vi "LVClass_WavefrontCorrectorSet ctor from WavefrontCorrector.vi"(0 "WavefrontCorrectorSet (const)":refnum<class "WavefrontCorrectorSet.lvclass">, 5 "WavefrontCorrectorSet":refnum<class "WavefrontCorrector.lvclass">, 11 "error in (no error)":errorcluster) -> (4 "WavefrontCorrectorSet (new)":refnum<class "WavefrontCorrectorSet.lvclass">, 6 "WavefrontCorrectorSet (dup)":refnum<class "WavefrontCorrector.lvclass">, 15 "error out":errorcluster)   [LabVIEW 2020, in "WavefrontCorrectorSet.lvclass"]
doc: "WavefrontCorrectorSet constructor.\n\n--------------------------------------------------------------------------------\n\n<B>wavefrontcorrector_setIn </B> : Constant Pointer to WavefrontCorrectorSet object.\n<B>wavefrontcorrector_setOut </B> : Constant Pointer to WavefrontCorrectorSet object.\n<B>config_file_path </B> : Absolute path to Haso or Camera configuration file.\n<B>ErrorIn </B> : Error\n<B>ErrorOut </B> : Error\n\n--------------------------------------------------------------------------------"
uses:
  WavefrontCorrectorSet.lvclass
  WavefrontCorrector.lvclass
  Handle creation.ctl
  WavefrontCorrectorSet.lvclass/WavefrontCorrectorSet.ctl
  LVClass_WavefrontCorrector Read WavefrontCorrector.vi
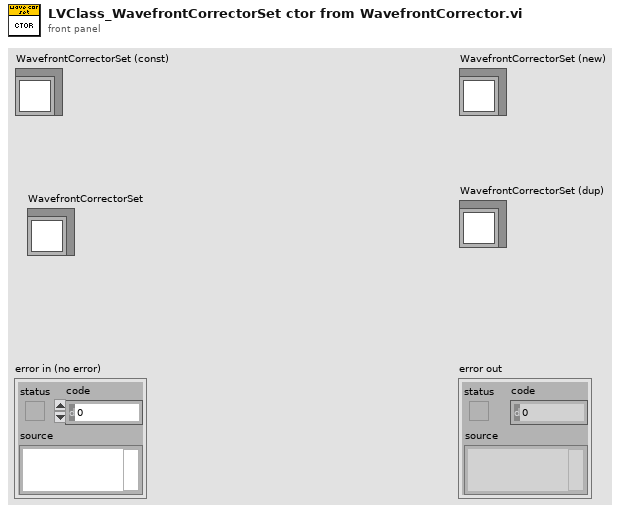
[diagram p1: front panel]
types:
  T1 = typedef "Handle creation.ctl" = enum16{"By ctor", "By write function"}
  T2 = typedef "ClassID.ctl" = i64
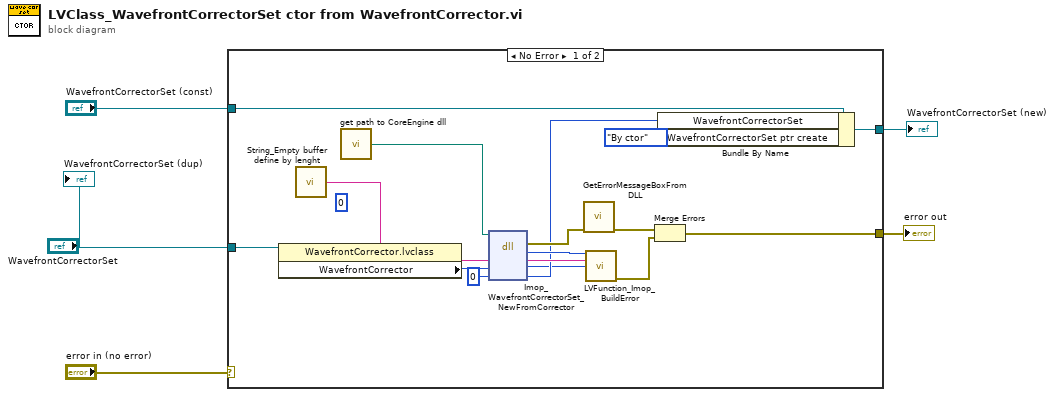
[diagram p0: block diagram]
diagram:
  n1 = case shown="No Error" "error in (no error)" {
    selector: "error in (no error)" -> [_ w23]
    tunnel: [w13 w23] -> w2
    tunnel: [w16 w22] -> w3
    tunnel: "WavefrontCorrectorSet (const)" -> [w17 w22]
    tunnel: "WavefrontCorrectorSet" -> [w11 _]
    frame No Error {
      (unwired) 0 ("Pupil")
      n2 = property class="WavefrontCorrector.lvclass"(reference=w11) -> ("WavefrontCorrector"=w9:T2)  [unwired: 1 in, 2 out]
      n3 = call "String_Empty buffer define by lenght.vi"() -> ("Empty buffer"=w10:string)  [unwired: 1 in]
      n4 = call "get path to CoreEngine dll.vi"() -> ("path to wavekit library"=w12:path)  [unwired: 14 in, 1 out]
      n5 = dll-call lib="D:/soft/HASO_v3/SVN_trunk/ImOpCoreEngine4_LV2011/DLLs/c_interface_vc100.dll" fn="Imop_WavefrontCorrectorSet_NewFromCorrector"(path in=w12, "message"=w10, "WavefrontCorrector"=w9, "WavefrontCorrectorSet"=i64 0) -> (error out=w19:errorcluster, "return type"=w20:i32, "message"=w21:string, "WavefrontCorrector"=w6:i64, "WavefrontCorrectorSet"=w8:i64)  [unwired: 2 in, 1 out]
      n6 = call "GetErrorMessageBoxFromDLL.vi"("error IN"=w19) -> ("error OUT"=w15:errorcluster)  [unwired: 10 in]
      n7 = call "LVFunction_Imop_BuildError.vi"("code"=w20, "String to Prepend to source (\"\")"=w21, "Adresse"=w6) -> ("error out"=w14:errorcluster)  [unwired: 12 in]
      n8 = Merge Errors(w15, w14) -> (w13:errorcluster)
      n9 = Bundle By Name(cluster=w17, "WavefrontCorrectorSet"=w8, "WavefrontCorrectorSet ptr create"=Handle_creation."By ctor" ("Pupil ptr create")) -> (w16:refnum<class "WavefrontCorrectorSet.lvclass">)
    }
    frame Error {
    }
  }
  "error out" <- w2
  "WavefrontCorrectorSet (new)" <- w3
  "WavefrontCorrectorSet (dup)" <- "WavefrontCorrectorSet"
